vi "Bracket a string.vi"(4 "String":string) -> (1 "<string>":string)   [LabVIEW 2013]
doc: "Prepends < and postpends > to a string."
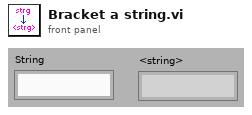
[diagram p1: front panel]
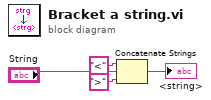
[diagram p0: block diagram]
diagram:
  n1 = Concatenate Strings("<" ("string"), "String", ">" ("string")) -> (→"<string>":string)
